vi "Add HTML Documentation for VI's parent item.vi"(11 "error in (no error)":errorcluster) -> (15 "error out":errorcluster)   [LabVIEW 2012]
doc: "VI Description text"
uses:
  _Controls and TypeDefs/InfoFromOldHTML_cluster.ctl
  _Controls and TypeDefs/StartPathLocation_enum.ctl
  _Controls and TypeDefs/UserDialogStates.ctl
  <vilib>/Platform/browser.llb/Open URL in Default Browser (string).vi
  <vilib>/Platform/browser.llb/Open URL in Default Browser (path).vi
panel:
  in  "www.labicom.net":bool
  in  "_vi_name_":string caption="Name"
  in  "Table":string[][](table)=[[" "]]
  in  "Help Button":bool
  out "LV <help> directory?":bool
  in  "Info extracted from old HTML":T1={"_vi_name_"="", "_vi_description_text_"="", "_vi_controls_and_indicators_descriptions_"="", "_name_of_owning_library_"="", "_owning_library_html_"="", "_Packages_"="Base Package", "_Platforms_"="Windows", "_details_text_"="Put details here", "_example_screenshot_"="", "_example_vi_"="", "_path_to_example_file_"=path "", "IsDetailsON?"=FALSE, "IsOwningLibraryON?"=FALSE, "IsExamplesON?"=FALSE, "IsTableON?"=FALSE, "IsScrollableON?"=FALSE, "IsDetailedHelpLinkON?"=FALSE, "Table Objects array"=[], "Table Descriptions array"=[], "Table Links array"=[], "Start path location"=enum."VI folder"}
  in  "Next_btn":bool
  out "HTML File Path":path
  in  "Cancel Button":bool
  out "Cancelled by User?":bool
  in  "Examples_chkBox":bool=TRUE
  in  "Details_chkBox":bool=TRUE
  in  "OwningLibrary_chkBox":bool=TRUE
  in  "Name of Owning Library":string="Put a name here" caption="Name of Owning Library or Palette"
  in  "Path to Owning Library":string caption="Path to Owning Library or Palette"
  in  "Names of Packages":string="Base Package" caption="Names of libraries/packages that this item requires for its operation"
  in  "Names of Platforms":string="Windows" caption="Names of platforms that this item supports"
  in  "Details":string="Put details here"
  in  "Image Path for Example":string caption="Path to the image file for Example category"
  in  "Example VI name":string
  in  "Example VI Path":path
  in  "VI Description":string caption="Item Description (with HTML tags)"
  in  "Start path location":enum32{"VI folder", "Help folder"}(radio)
  in  "Documentable VI Path":path
  # "Configure parent item Documentation Layout"
  # "Additional layout elements for LabVIEW help"
  # "Caution: place <_caution_> into your text"
  # "Note: place <_note_> into your text"
  # "Tip: place <_tip_> into your text"
  # "Windows"
  # "Platform: enclose platform name between\n<_platform_> and </_platform_> tags"
  # "bold"
  # "Text in bold: enclose such text between\n<B> and </B> tags"
  # "Attention!"
  # "Caution Text: enclose such text between \n<_caution_text_> and </_caution_text_> tags"
  # "vigods.com"
  # "Link: place path in place of '_path_' and text in \nplace of '_text_' and insert resulting string\nwherever you need: \n<a href=\"_path_\">_text_</a>"
  # "monospace"
  # "Monospace: enclose such text between\n<_monospace_> and </_monospace_> tags"
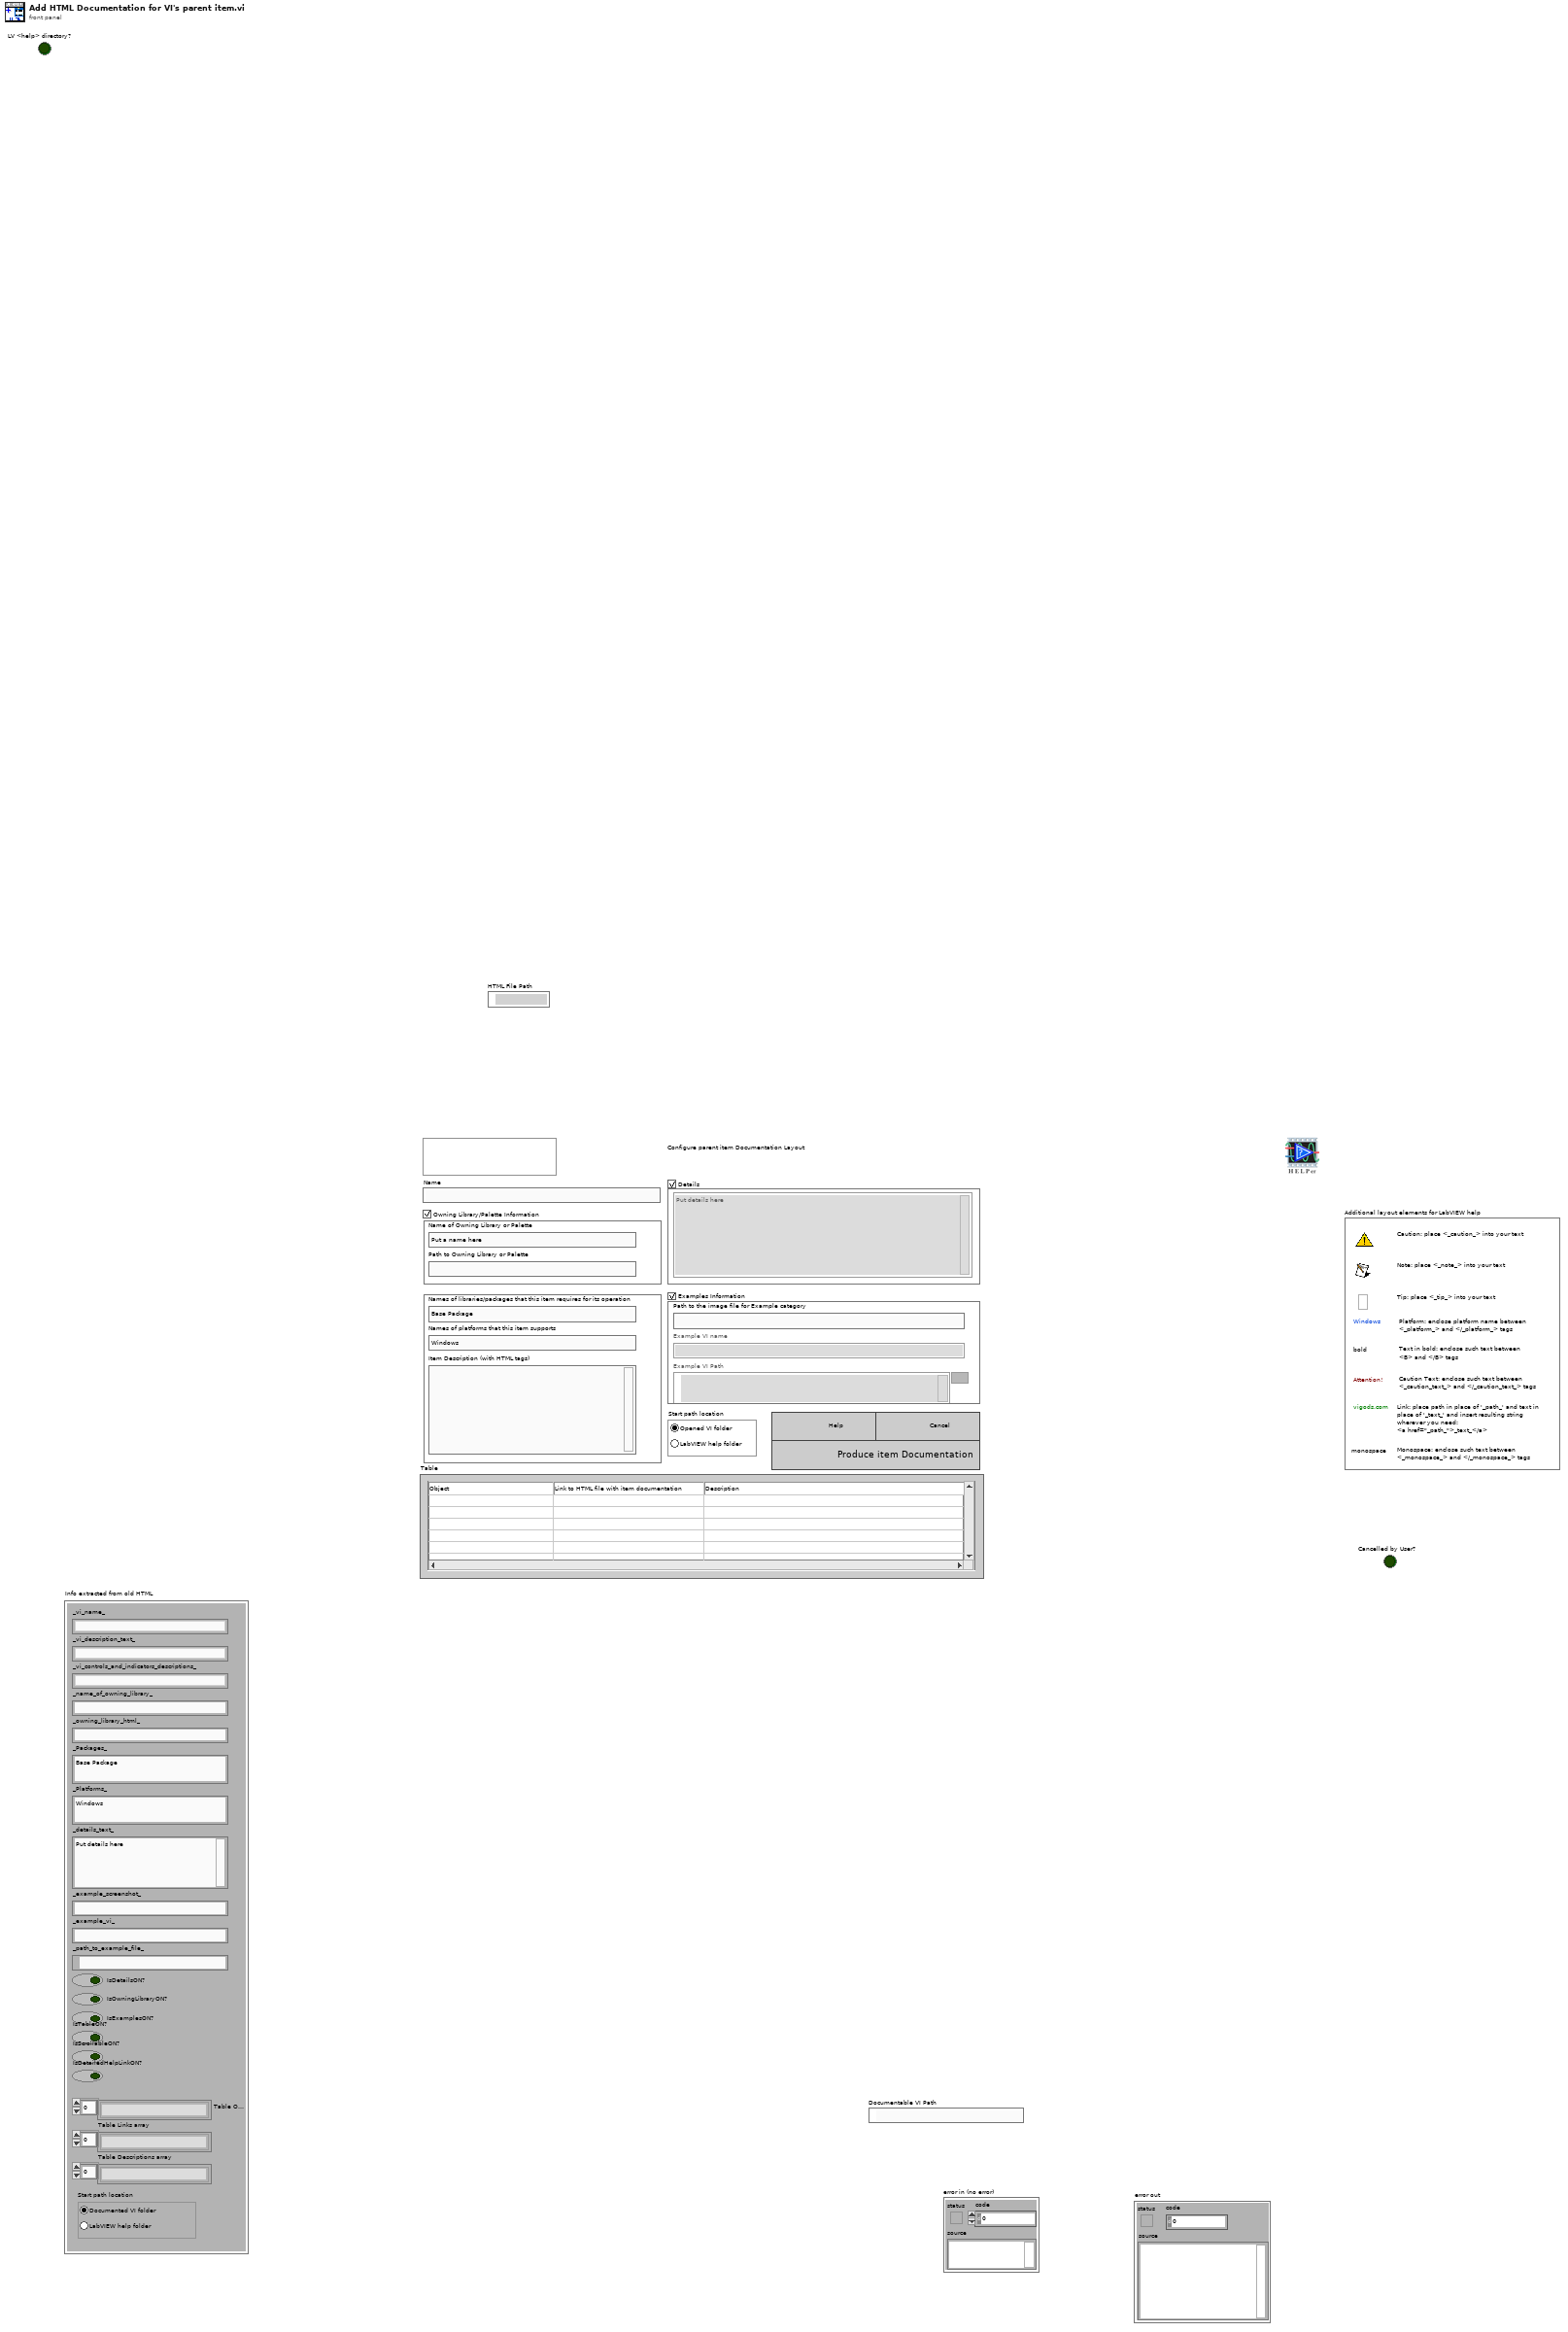
[diagram p1: front panel]
types:
  T1 = typedef "InfoFromOldHTML_cluster.ctl" = cluster{"_vi_name_":string, "_vi_description_text_":string, "_vi_controls_and_indicators_descriptions_":string, "_name_of_owning_library_":string, "_owning_library_html_":string, "_Packages_":string, "_Platforms_":string, "_details_text_":string, "_example_screenshot_":string, "_example_vi_":string, "_path_to_example_file_":path, "IsDetailsON?":bool, "IsOwningLibraryON?":bool, "IsExamplesON?":bool, "IsTableON?":bool, "IsScrollableON?":bool, "IsDetailedHelpLinkON?":bool, "Table Objects array":string[], "Table Descriptions array":string[], "Table Links array":string[], "Start path location":T2}
  T2 = typedef "StartPathLocation_enum.ctl" = enum32{"VI folder", "Help folder"}
  T3 = typedef "UserDialogStates.ctl" = enum16{"Overview", "Known Issues", "Choose parameters", "Update", "Choose HTML file path", "Choose Images directory path", "Decide if there is Context Help", "Choose help hierarchy", "Generate HTML", "Installation", "System Requirements", "Software Support", "Device Support", "Upgrade Issues", "New Features", "Fixed Issues", "Developer", "Contact Support", "Copyright", "Trademarks", "Patents", "Disclaimer", "Save", "Shutdown"}
  T4 = enum8{"Enabled", "Disabled", "Disabled and Grayed Out"}
  T5 = typedef "LVRowAndColumnTypeDef.ctl" = cluster{"Row":i32, "Column":i32}
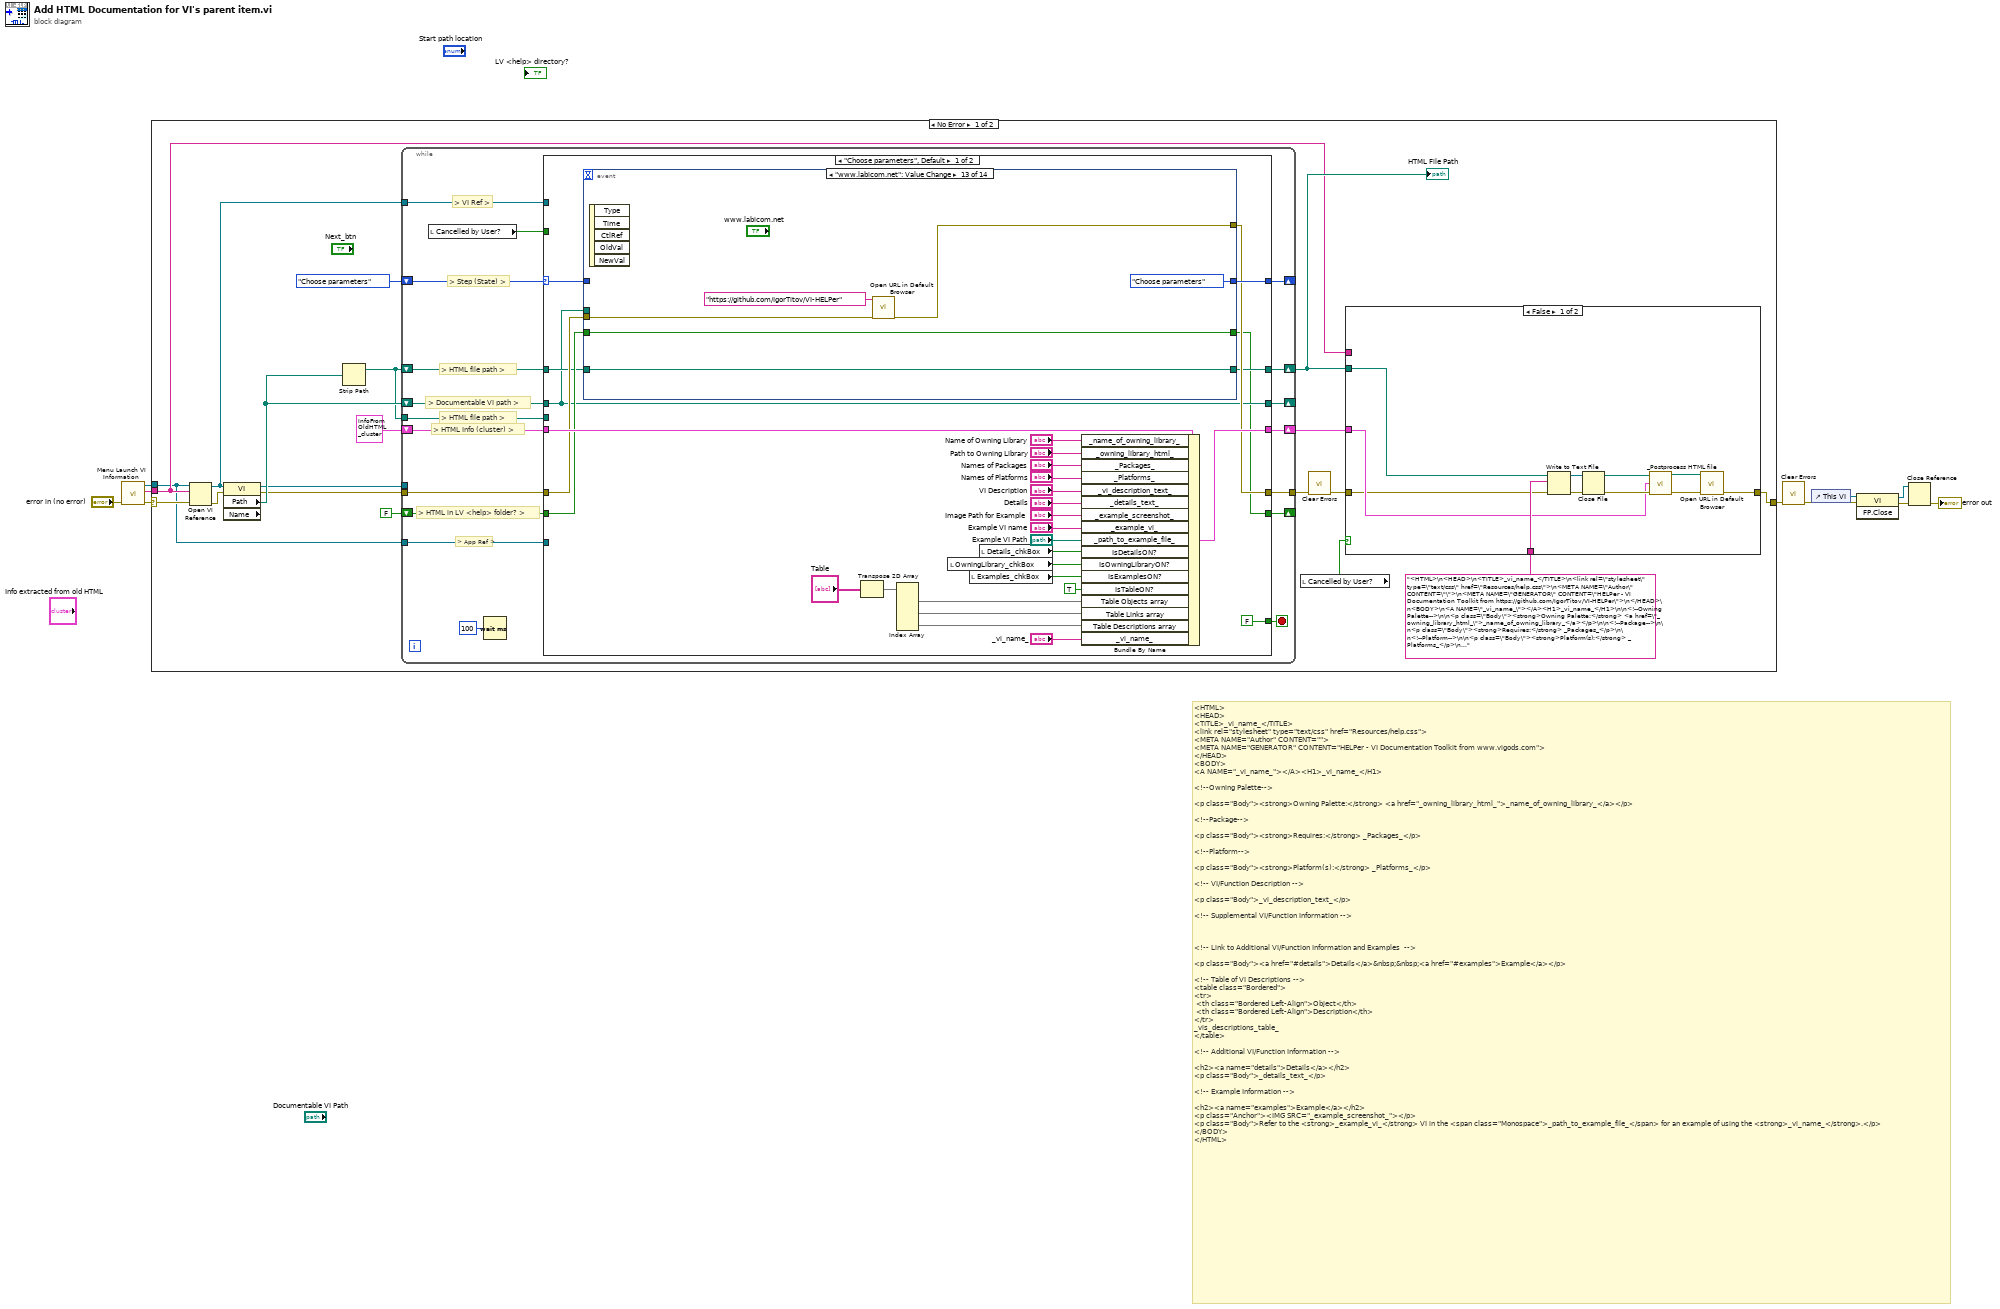
[diagram p0: block diagram]
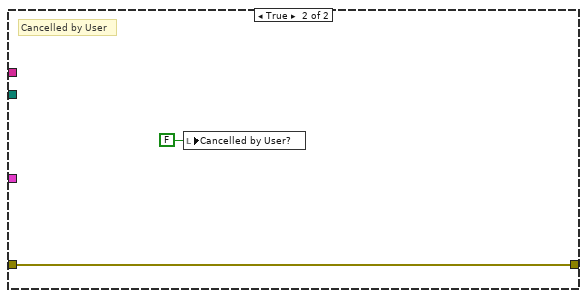
[diagram p2: hidden frame]
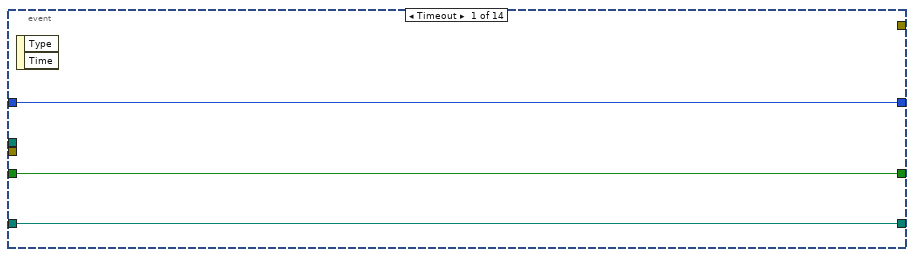
[diagram p3: hidden frame]
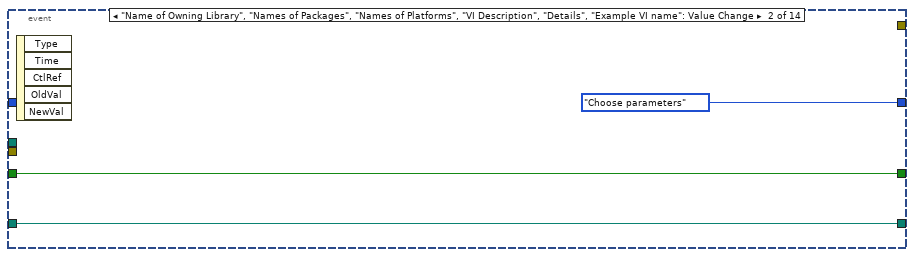
[diagram p4: hidden frame]
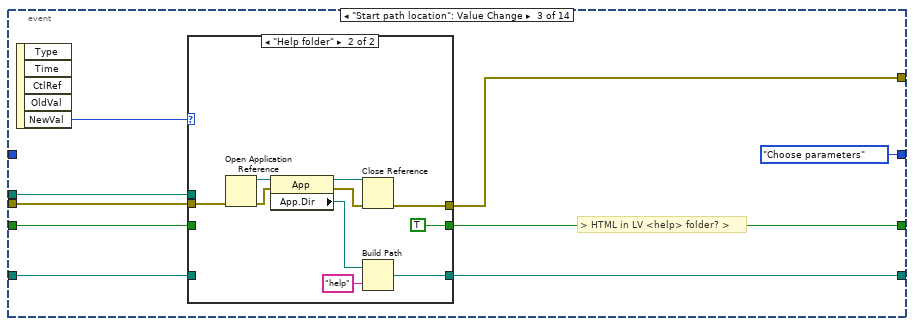
[diagram p5: hidden frame]
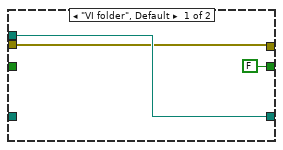
[diagram p6: hidden frame]
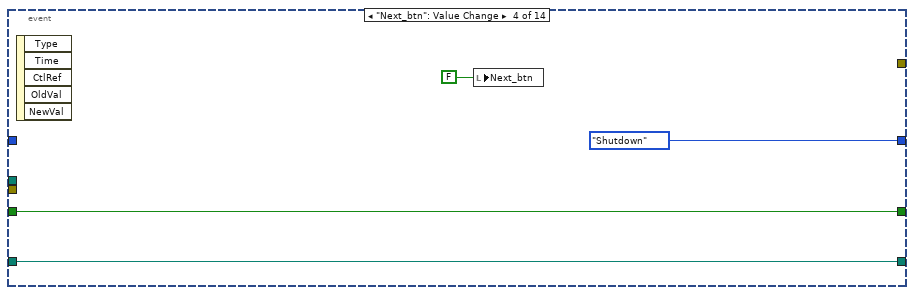
[diagram p7: hidden frame]
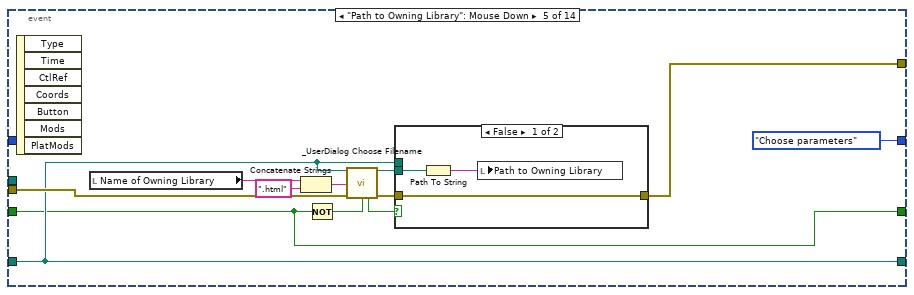
[diagram p8: hidden frame]
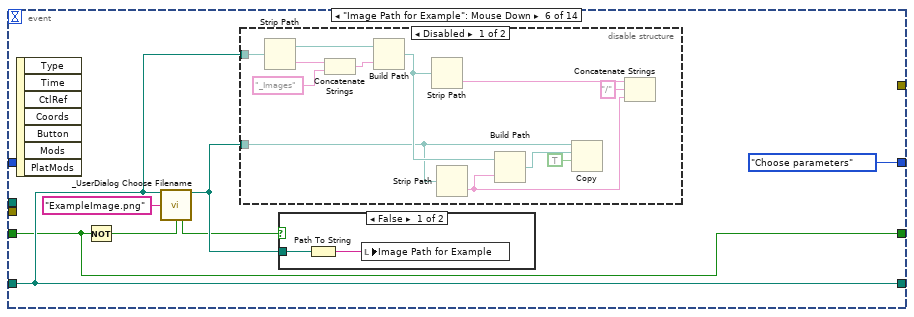
[diagram p10: hidden frame]
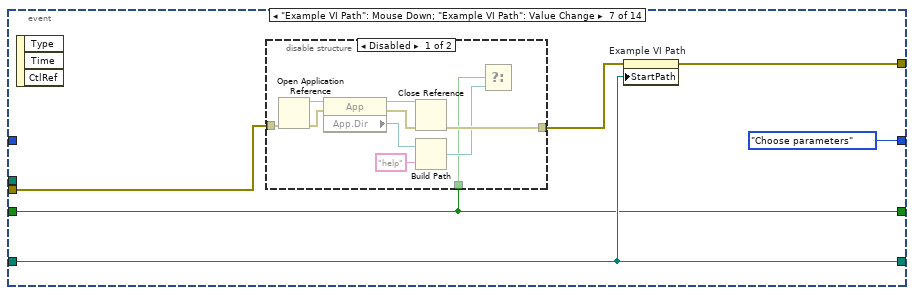
[diagram p13: hidden frame]
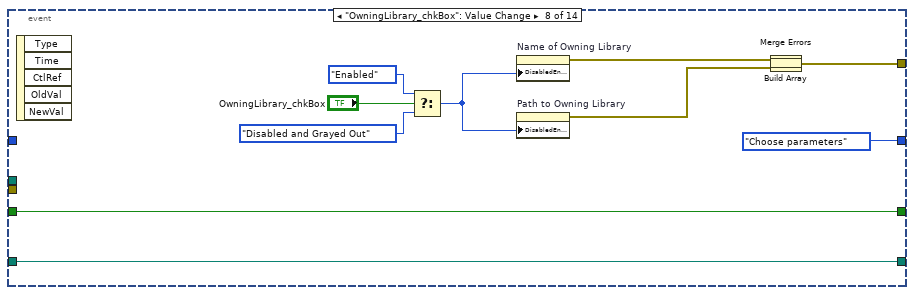
[diagram p15: hidden frame]
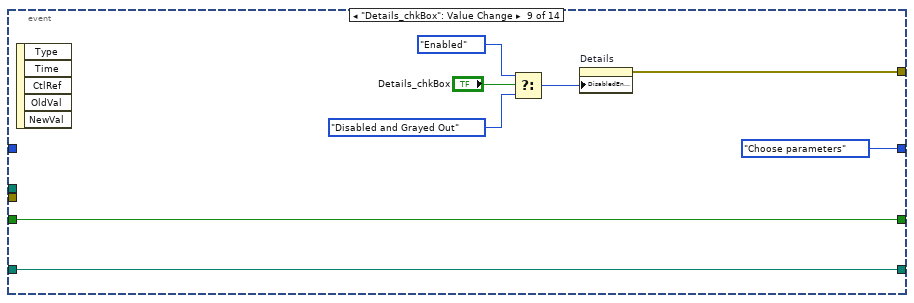
[diagram p16: hidden frame]
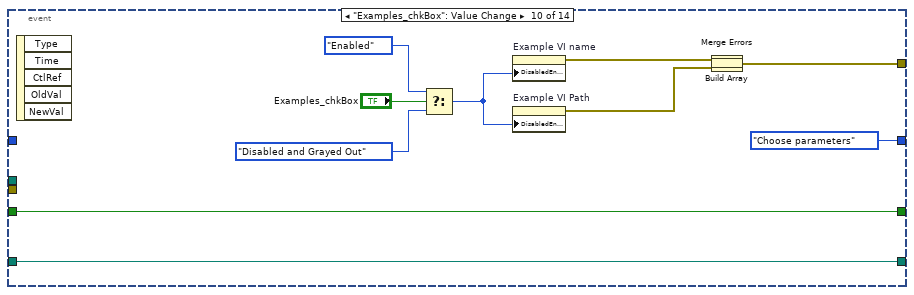
[diagram p17: hidden frame]
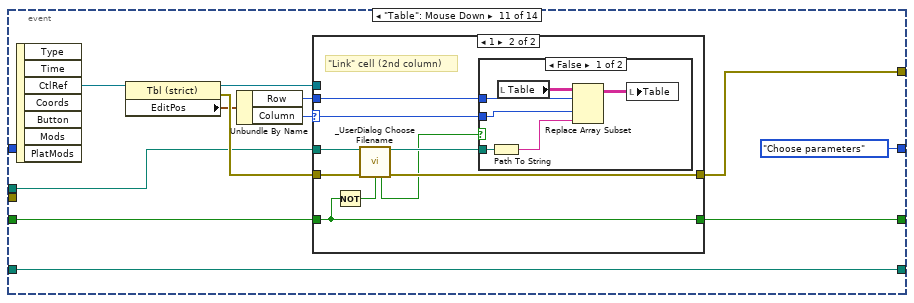
[diagram p18: hidden frame]
diagram:
  # "<HTML>\n<HEAD>\n<TITLE>_vi_name_</TITLE>\n<link rel=\"stylesheet\" type=\"text/css\" href=\"Resources/help.css\">\n<META NAME=\"Author\" CONTENT=\"\">\n<META NAME=\"GENERATOR\" CONTENT=\"HELPer - VI Documentation Toolkit from www.vigods.com\">\n</HEAD>\n<BODY>\n<A NAME=\"_vi_name_\"></A><H1>_vi_name_</H1>\n\n<!--Owning Palette-->\n\n<p class=\"Body\"><strong>Owning Palette:</strong> <a href=\"_owning_library_html_\">_name_of_owning_library_</a></p>\n\n<!--Package-->\n\n<p class=\"Body\"><strong>Requires:</strong> _Packages_</p>\n\n<!--Platform-->\n\n<p class=\"Body\"><strong>Platform(s):</strong> _Platforms_</p>\n\n<!-- VI/Function Description -->\n\n<p class=\"Body\">_vi_description_text_</p>\n\n<!-- Supplemental VI/Function Information -->\n\n\n\n<!-- Link to Additional VI/Function Information and Examples  -->\n\n<p class=\"Body\"><a href=\"#details\">Details</a>&nbsp;&nbsp;<a href=\"#examples\">Example</a></p>\n\n<!-- Table of VI Descriptions -->\n<table class=\"Bordered\">\n<tr>\n\t<th class=\"Bordered Left-Align\">Object</th>\n\t<th class=\"Bordered Left-Align\">Description</th>\n</tr>\n_vis_descriptions_table_\n</table>\n\n<!-- Additional VI/Function Information -->\n\n<h2><a name=\"details\">Details</a></h2>\n<p class=\"Body\">_details_text_</p>\n\n<!-- Example Information -->\n\n<h2><a name=\"examples\">Example</a></h2>\n<p class=\"Anchor\"><IMG SRC=\"_example_screenshot_\"></p>\n<p class=\"Body\">Refer to the <strong>_example_vi_</strong> VI in the <span class=\"Monospace\">_path_to_example_file_</span> for an example of using the <strong>_vi_name_</strong>.</p>\n</BODY>\n</HTML>"
  n1 = call <vilib>:"Menu Launch VI Information.vi"("error in (no error)"="error in (no error)") -> ("error out"=w7:errorcluster, "Menu Launch:VI"=w9:string, "Menu Launch:App"=w10:refnum<vi>)  [unwired: 8 in]
  n2 = case shown="No Error" w7 {
    selector: w7 -> [w26 w350]
    tunnel: w10 -> [w17 _]
    tunnel: w9 -> [w18 _]
    tunnel: [w23 w350] -> w2
    frame No Error {
      n3 = Open VI Reference(application reference (local)=w17, vi path=w18, error in (no error)=w26) -> (vi reference=w19:refnum<vi>, error out=w29:errorcluster)  [unwired: 3 in]
      n4 = property class="VI" props=["Path", "Name"](reference=w19, error in=w29) -> (reference out=w15:refnum<vi>, error out=w16:errorcluster, "Path"=w21:path)  [unwired: 1 out]
      n5 = Strip Path(path=w21) -> (stripped path=w20:path)  [unwired: 1 out]
      n6 = while {
        shift-right: [w57] -> _
        shift-left: UserDialogStates."Choose parameters" ("UserDialogSteps") -> [w58]
        tunnel: w20 -> [w56]
        shift-right: [w55] -> w22
        shift-left: w20 -> [w54]
        shift-right: [w52] -> w24
        shift-left: T1 {"_vi_name_"="", "_vi_description_text_"="", "_vi_controls_and_indicators_descriptions_"="", "_name_of_owning_library_"="", "_owning_library_html_"="", "_Packages_"="Base Package", "_Platforms_"="Windows", "_details_text_"="Put details here", "_example_screenshot_"="", "_example_vi_"="", "_path_to_example_file_"=path "", "IsDetailsON?"=FALSE, "IsOwningLibraryON?"=FALSE, "IsExamplesON?"=FALSE, "IsTableON?"=FALSE, "IsScrollableON?"=FALSE, "IsDetailedHelpLinkON?"=FALSE, "Table Objects array"=[], "Table Descriptions array"=[], "Table Links array"=[], "Start path location"=enum."VI folder"} ("Info extracted from old HTML") -> [w53]
        tunnel: w16 -> [w50]
        shift-right: [w47] -> _
        shift-left: FALSE -> [w51]
        shift-right: [w46] -> _
        shift-left: w21 -> [w49]
        tunnel: [w48] -> w12
        tunnel: w19 -> [w44]
        tunnel: w17 -> [w43]
        tunnel: w15 -> [_]
        stop <- w60 stop-if-true
        # "> App Ref >"
        # "> VI Ref >"
        # "> Documentable VI path >"
        # "> HTML file path >"
        # "> HTML in LV <help> folder? >"
        # "> HTML Info (cluster) >"
        # "> Step (State) >"
        # "> HTML file path >"
        n7 = local read "Cancelled by User?"() -> (w45:bool)
        n8 = Wait (ms)(milliseconds to wait=u32 100) -> ()  [unwired: 1 out]
        n9 = case shown="\"Choose parameters\", Default" w58 {
          selector: w58 -> [w90 w256]
          tunnel: [FALSE w269] -> w60
          tunnel: [w89 w262] -> w57
          tunnel: w56 -> [_ _]
          tunnel: [w70 w260] -> w55
          tunnel: w54 -> [w71 w263]
          tunnel: w53 -> [w88 w266]
          tunnel: [w78 w265] -> w52
          tunnel: w51 -> [w72 w259]
          tunnel: w50 -> [w74 w268]
          tunnel: w49 -> [w69 w267]
          tunnel: [w73 w264] -> w48
          tunnel: [w68 w258] -> w47
          tunnel: [w69 w261] -> w46
          tunnel: w45 -> [_ w257]
          tunnel: w44 -> [_ w255]
          tunnel: w43 -> [_ w254]
          frame "Choose parameters", Default {
            n10 = event shown="[12] \"www.labicom.net\": Value Change" {
              selector: _ -> [_ _ _ _ _ _ _ _ _ _ _ _ _ _]
              dyn-events: _ -> [_ _ _ _ _ _ _ _ _ _ _ _ _ _]
              timeout: _ -> [_ _ _ _ _ _ _ _ _ _ _ _ _ _]
              tunnel: w90 -> [w94 _ _ _ _ _ _ _ _ _ _ _ _ _]
              tunnel: [w94 UserDialogStates."Choose parameters" ("UserDialogSteps") UserDialogStates."Choose parameters" ("UserDialogSteps") UserDialogStates."Shutdown" ("UserDialogSteps") UserDialogStates."Choose parameters" ("UserDialogSteps") UserDialogStates."Choose parameters" ("UserDialogSteps") UserDialogStates."Choose parameters" ("UserDialogSteps") UserDialogStates."Choose parameters" ("UserDialogSteps") UserDialogStates."Choose parameters" ("UserDialogSteps") UserDialogStates."Choose parameters" ("UserDialogSteps") UserDialogStates."Choose parameters" ("UserDialogSteps") UserDialogStates."Choose parameters" ("UserDialogSteps") UserDialogStates."Choose parameters" ("UserDialogSteps") UserDialogStates."Shutdown" ("UserDialogSteps")] -> w89
              tunnel: w72 -> [w92 w95 w99 w120 w124 w140 w161 w179 w189 w198 w213 w241 w244 w249]
              tunnel: w74 -> [_ _ w102 _ w129 _ w164 _ _ _ _ w238 w247 w252]
              tunnel: [_ _ w101 _ w128 _ w163 w180 w191 w200 w211 w237 w246 w252] -> w73
              tunnel: w71 -> [w93 w96 w104 w121 w127 w144 w162 w183 w190 w199 w212 w240 w245 w250]
              tunnel: [w93 w96 w103 w121 w127 w144 w162 w183 w190 w199 w212 w240 w245 w250] -> w70
              tunnel: w69 -> [_ _ w100 _ _ _ _ _ _ _ w214 _ _ _]
              tunnel: [w92 w95 w98 w120 w124 w140 w161 w179 w189 w198 w208 w241 w244 w249] -> w68
              event Timeout {
                n11 = event-data() -> ()  [unwired: 1 in, 2 out]
              }
              event "Name of Owning Library", "Names of Packages", "Names of Platforms", "VI Description", "Details", "Example VI name": Value Change {
                n12 = event-data() -> ()  [unwired: 1 in, 5 out]
              }
              event "Start path location": Value Change {
                # "> HTML in LV <help> folder? >"
                n13 = event-data() -> ("NewVal"=w105:enum32{"VI folder", "Help folder"})  [unwired: 1 in, 4 out]
                n14 = case shown="\"Help folder\"" w105 {
                  tunnel: w104 -> [_ _]
                  tunnel: [w109 w113] -> w103
                  tunnel: w102 -> [w108 w112]
                  tunnel: [w108 w111] -> w101
                  tunnel: w100 -> [w109 _]
                  tunnel: w99 -> [_ _]
                  tunnel: [FALSE TRUE] -> w98
                  frame "VI folder", Default {
                  }
                  frame "Help folder" {
                    n15 = Open Application Reference(8:w112) -> (0:w115:errorcluster, 3:w114:refnum<vi>)  [unwired: 3 in]
                    n16 = property class="App"(reference=w114, error in=w115) -> (reference out=w116:refnum<vi>, error out=w117:errorcluster, "App.Dir"=w118:path)
                    n17 = Close Reference(reference=w116, error in (no error)=w117) -> (error out=w111:errorcluster)
                    n18 = Build Path(base path=w118, name or relative path="help") -> (appended path=w113:path)
                  }
                }
              }
              event "Next_btn": Value Change {
                n19 = event-data() -> ()  [unwired: 1 in, 5 out]
                n20 = local write "Next_btn"(FALSE ("Next Button")) -> ()
              }
              event "Path to Owning Library": Mouse Down {
                n21 = event-data() -> ()  [unwired: 1 in, 7 out]
                n22 = local read "Name of Owning Library"() -> (w134:string)
                n23 = Concatenate Strings(w134, ".html" ("string")) -> (w133:string)
                n24 = Not(x=w124) -> (.not. x?=w125:bool)
                n25 = call "_UserDialog Choose Filename.vi"("VI Default Path"=w127, "Default file name"=w133, "error in (no error)"=w129, "Not In <help> directory? (Yes: T)"=w125) -> ("HTML File Path"=w131:path, "Cancelled by User?"=w126:bool, "error out"=w130:errorcluster)  [unwired: 7 in, 2 out]
                n26 = case shown="False" w126 {
                  tunnel: w131 -> [w138 _]
                  tunnel: w130 -> [w136 w139]
                  tunnel: [w136 w139] -> w128
                  tunnel: w127 -> [_ _]
                  frame False {
                    n27 = Path To String(path=w138) -> (string=w137:string)
                    n28 = local write "Path to Owning Library"(w137) -> ()
                  }
                  frame True {
                  }
                }
              }
              event "Image Path for Example": Mouse Down {
                n29 = event-data() -> ()  [unwired: 1 in, 7 out]
                n30 = Not(x=w140) -> (.not. x?=w141:bool)
                n31 = call "_UserDialog Choose Filename.vi"("VI Default Path"=w144, "Default file name"="ExampleImage.png", "Not In <help> directory? (Yes: T)"=w141) -> ("HTML File Path"=w143:path, "Cancelled by User?"=w142:bool)  [unwired: 8 in, 3 out]
                n32 = disable-structure shown="Disabled" {
                  disable-tunnel: w144 -> [w148 _]
                  disable-tunnel: w143 -> [w147 _]
                  frame Disabled {
                    n33 = Strip Path(path=w148) -> (stripped path=w150:path, name=w152:string)
                    n34 = Concatenate Strings(w152, "_Images" ("name or relative path")) -> (w153:string)
                    n35 = Build Path(base path=w150, name or relative path=w153) -> (appended path=w149:path)
                    n36 = Strip Path(path=w149) -> (name=w156:string)  [unwired: 1 out]
                    n37 = Strip Path(path=w147) -> (name=w155:string)  [unwired: 1 out]
                    n38 = Build Path(base path=w149, name or relative path=w155) -> (appended path=w158:path)
                    n39 = Copy(9:TRUE ("overwrite (F)"), 10:w158, 11:w147) -> ()  [unwired: 2 in, 3 out]
                    n40 = Concatenate Strings(w156, "/" ("string"), w155) -> ()  [unwired: 1 out]
                  }
                  frame Enabled {
                  }
                }
                n41 = case shown="False" w142 {
                  tunnel: w143 -> [w160 _]
                  frame False {
                    n42 = Path To String(path=w160) -> (string=w159:string)
                    n43 = local write "Image Path for Example"(w159) -> ()
                  }
                  frame True {
                  }
                }
              }
              event "Example VI Path": Mouse Down; "Example VI Path": Value Change {
                n44 = event-data() -> ()  [unwired: 1 in, 3 out]
                n45 = disable-structure shown="Disabled" {
                  disable-tunnel: [w176 w177] -> w165
                  disable-tunnel: w161 -> [w168 _]
                  disable-tunnel: w164 -> [w167 w177]
                  frame Disabled {
                    n46 = Open Application Reference(8:w167) -> (0:w173:errorcluster, 3:w174:refnum<vi>)  [unwired: 3 in]
                    n47 = property class="App"(reference=w174, error in=w173) -> (reference out=w172:refnum<vi>, error out=w171:errorcluster, "App.Dir"=w170:path)
                    n48 = Close Reference(reference=w172, error in (no error)=w171) -> (error out=w176:errorcluster)
                    n49 = Build Path(base path=w170, name or relative path="help") -> (appended path=w175:path)
                    n50 = Select(s=w168, f=w175) -> ()  [unwired: 1 in, 1 out]
                  }
                  frame Enabled {
                  }
                }
                n51 = property on="Example VI Path" class="Path"(error in=w165, "StartPath"=w162) -> (error out=w163:errorcluster)  [unwired: 1 in, 1 out]
              }
              event "OwningLibrary_chkBox": Value Change {
                n52 = event-data() -> ()  [unwired: 1 in, 5 out]
                n53 = Select(t=T4."Enabled" ("Disabled"), s="OwningLibrary_chkBox", f=T4."Disabled and Grayed Out") -> (s? t:f=w184:T4)
                n54 = property on="Name of Owning Library" class="Str"("DisabledEnum"=w184) -> (error out=w182:errorcluster)  [unwired: 2 in, 1 out]
                n55 = property on="Path to Owning Library" class="Str"("DisabledEnum"=w184) -> (error out=w181:errorcluster)  [unwired: 2 in, 1 out]
                n56 = Build Array(w182, w181) -> (w178:errorcluster[])
                n57 = Merge Errors(w178) -> (w180:errorcluster)
              }
              event "Details_chkBox": Value Change {
                n58 = event-data() -> ()  [unwired: 1 in, 5 out]
                n59 = Select(t=T4."Enabled" ("Disabled"), s="Details_chkBox", f=T4."Disabled and Grayed Out") -> (s? t:f=w194:T4)
                n60 = property on="Details" class="Str"("DisabledEnum"=w194) -> (error out=w191:errorcluster)  [unwired: 2 in, 1 out]
              }
              event "Examples_chkBox": Value Change {
                n61 = event-data() -> ()  [unwired: 1 in, 5 out]
                n62 = Select(t=T4."Enabled" ("Disabled"), s="Examples_chkBox", f=T4."Disabled and Grayed Out") -> (s? t:f=w204:T4)
                n63 = property on="Example VI name" class="Str"("DisabledEnum"=w204) -> (error out=w202:errorcluster)  [unwired: 2 in, 1 out]
                n64 = property on="Example VI Path" class="Path"("DisabledEnum"=w204) -> (error out=w201:errorcluster)  [unwired: 2 in, 1 out]
                n65 = Build Array(w202, w201) -> (w197:errorcluster[])
                n66 = Merge Errors(w197) -> (w200:errorcluster)
              }
              event "Table": Mouse Down {
                n67 = event-data() -> ("CtlRef"=w210:refnum<vi>)  [unwired: 1 in, 6 out]
                n68 = property class="Tbl (strict)"(reference=w210) -> (reference out=w217:refnum<vi>, error out=w218:errorcluster, "EditPos"=w215:T5)  [unwired: 1 in]
                n69 = Unbundle By Name(w215) -> ("Row"=w219:i32, "Column"=w216:i32)
                n70 = case shown="1" w216 {
                  selector: w216 -> [_ w226]
                  tunnel: w213 -> [w220 w224]
                  tunnel: w214 -> [_ w230]
                  tunnel: w217 -> [_ _]
                  tunnel: w218 -> [w221 w228]
                  tunnel: w219 -> [_ w227]
                  tunnel: [w221 w225] -> w211
                  tunnel: [w220 w224] -> w208
                  frame 0, Default {
                  }
                  frame 1 {
                    # "\"Link\" cell (2nd column)"
                    n71 = Not(x=w224) -> (.not. x?=w223:bool)
                    n72 = call "_UserDialog Choose Filename.vi"("VI Default Path"=w230, "error in (no error)"=w228, "Not In <help> directory? (Yes: T)"=w223) -> ("HTML File Path"=w229:path, "Cancelled by User?"=w222:bool, "error out"=w225:errorcluster)  [unwired: 8 in, 2 out]
                    n73 = case shown="False" w222 {
                      tunnel: w229 -> [w236 _]
                      tunnel: w227 -> [w234 _]
                      tunnel: w226 -> [w233 _]
                      frame False {
                        n74 = Path To String(path=w236) -> (string=w232:string)
                        n75 = local read "Table"() -> (w235:string[][])
                        n76 = Replace Array Subset(array=w235, new element=w232, index (row)=w234, index (col)=w233) -> (w231:string[][])
                        n77 = local write "Table"(w231) -> ()
                      }
                      frame True {
                      }
                    }
                  }
                }
              }
              event "Help Button": Value Change {
                n78 = event-data() -> ()  [unwired: 1 in, 5 out]
                n79 = call "Read me and Help.vi"("path"=path "viGods.com/HELPer/parent.html", "error in"=w238) -> ("error out"=w237:errorcluster)  [unwired: 13 in]
              }
              event "www.labicom.net": Value Change {
                n80 = event-data() -> ()  [unwired: 1 in, 5 out]
                n81 = call-poly <vilib>:"Open URL in Default Browser.vi"("error in (no error)"=w247, "URL"="https://github.com/IgorTitov/VI-HELPer") -> ("error out"=w246:errorcluster)  [unwired: 4 in, 1 out]
              }
              event "Cancel Button": Value Change {
                n82 = event-data() -> ()  [unwired: 1 in, 5 out]
                "Cancelled by User?" <- TRUE ("Cancelled by User?")
              }
            }
            n83 = Transpose 2D Array(2D array="Table") -> (transposed array=w62:string[][])
            n84 = Index Array(array=w62) -> (element #1=w66:string[], element #2=w65:string[], element #3=w64:string[])  [unwired: 6 in]
            n85 = local read "OwningLibrary_chkBox"() -> (w76:bool)
            n86 = local read "Examples_chkBox"() -> (w75:bool)
            n87 = local read "Details_chkBox"() -> (w77:bool)
            n88 = Bundle By Name(cluster=w88, "_name_of_owning_library_"="Name of Owning Library", "_owning_library_html_"="Path to Owning Library", "_Packages_"="Names of Packages", "_Platforms_"="Names of Platforms", "_vi_description_text_"="VI Description", "_details_text_"="Details", "_example_screenshot_"="Image Path for Example", "_example_vi_"="Example VI name", "_path_to_example_file_"="Example VI Path", "IsDetailsON?"=w77, "IsOwningLibraryON?"=w76, "IsExamplesON?"=w75, "IsTableON?"=TRUE, "Table Objects array"=w66, "Table Links array"=w65, "Table Descriptions array"=w64, "_vi_name_"="_vi_name_") -> (w78:T1)
          }
          frame "Shutdown" {
            n89 = case shown="False" w257 {
              tunnel: [w289 TRUE] -> w269
              tunnel: w268 -> [w288 w342]
              tunnel: w267 -> [w287 w345]
              tunnel: w266 -> [w286 w346]
              tunnel: [w285 w346] -> w265
              tunnel: [w284 w341] -> w264
              tunnel: w263 -> [w283 w344]
              tunnel: [w281 UserDialogStates."Shutdown" ("UserDialogSteps")] -> w262
              tunnel: [w280 w345] -> w261
              tunnel: [w279 w344] -> w260
              tunnel: w259 -> [w276 w347]
              tunnel: [w277 w347] -> w258
              tunnel: w256 -> [_ _]
              tunnel: w255 -> [w272 w343]
              tunnel: w254 -> [w271 _]
              frame False {
                # "> VI Name >"
                n90 = Concatenate Strings("parent_item" ("string"), ".html" ("string")) -> (w273:string)
                n91 = Not(x=w276) -> (.not. x?=w275:bool)
                n92 = call "_UserDialog Choose Filename.vi"("VI Default Path"=w283, "Default file name"=w273, "Not In <help> directory? (Yes: T)"=w275) -> ("HTML File Path"=w282:path, "Cancelled by User?"=w278:bool)  [unwired: 8 in, 3 out]
                n93 = case shown="False" w278 {
                  tunnel: [TRUE FALSE] -> w289
                  tunnel: w288 -> [w293 w338]
                  tunnel: w287 -> [w302 w335]
                  tunnel: w286 -> [w317 w336]
                  tunnel: [w315 w336] -> w285
                  tunnel: [w313 w338] -> w284
                  tunnel: w282 -> [w295 w334]
                  tunnel: [UserDialogStates."Shutdown" ("UserDialogSteps") UserDialogStates."Choose parameters" ("UserDialogSteps")] -> w281
                  tunnel: [w302 w335] -> w280
                  tunnel: [w295 w334] -> w279
                  tunnel: w276 -> [w303 w337]
                  tunnel: [w303 w337] -> w277
                  tunnel: w272 -> [w298 _]
                  tunnel: w271 -> [_ _]
                  frame False {
                    # "Copy example image from location chosen by user\nto images folder of this HTML"
                    # "> HTML file path >"
                    # "> Documented VI path >"
                    # "> HTML file path >"
                    n94 = Unbundle By Name(w317) -> ("_owning_library_html_"=w323:string, "_example_screenshot_"=w307:string, "Table Links array"=w301:string[])
                    n95 = call "_Create HTML folders.vi"("HTML File Path"=w295, "error in (no error)"=w293) -> ("HTML Images Folder"=w292:path, "error out"=w294:errorcluster)  [unwired: 10 in, 2 out]
                    n96 = String To Path(string=w323) -> (path=w318:path)
                    n97 = String To Path(string=w307) -> (path=w306:path)
                    n98 = String To Path(string=w301) -> (path=w300:path[])
                    n99 = for {
                      tunnel: w300 -> [w328] mode=indexing
                      tunnel: w295 -> [w329]
                      tunnel: [w325] -> w299 mode=indexing
                      tunnel: w294 -> [w326]
                      tunnel: [w327] -> w296
                      n100 = call <vilib>:"Compare Two Paths.vi"("error in (no error)"=w326, "Path 2"=w328, "Path 1"=w329) -> ("error out"=w330:errorcluster, "Relative Path from 1 to 2"=w331:path)  [unwired: 5 in, 2 out]
                      n101 = Path To String(path=w331) -> (string=w332:string)
                      n102 = Search and Replace String(input string=w332, search string="..\\", error in=w330) -> (result string=w325:string, error out=w327:errorcluster)  [unwired: 5 in, 2 out]
                    }
                    n103 = call <vilib>:"Compare Two Paths.vi"("error in (no error)"=w294, "Path 2"=w318, "Path 1"=w295) -> ("error out"=w322:errorcluster, "Relative Path from 1 to 2"=w321:path)  [unwired: 5 in, 2 out]
                    n104 = Path To String(path=w321) -> (string=w320:string)
                    n105 = Strip Path(path=w306) -> (name=w311:string)  [unwired: 1 out]
                    n106 = Strip Path(path=w292) -> (name=w310:string)  [unwired: 1 out]
                    n107 = Search and Replace String(input string=w320, search string="..\\", error in=w322) -> (result string=w316:string, error out=w297:errorcluster)  [unwired: 5 in, 2 out]
                    n108 = Build Path(base path=w292, name or relative path=w311) -> (appended path=w308:path)
                    n109 = Copy(8:w297, 9:TRUE ("overwrite (F)"), 10:w308, 11:w306) -> (0:w291:errorcluster)  [unwired: 1 in, 2 out]
                    n110 = Concatenate Strings(w310, "/" ("string"), w311) -> (w305:string)
                    n111 = Bundle By Name(cluster=w317, "_owning_library_html_"=w316, "_example_screenshot_"=w305, "Table Links array"=w299) -> (w315:T1)
                    n112 = Close Reference(reference=w298, error in (no error)=w297) -> (error out=w314:errorcluster)
                    n113 = Build Array(w314, w296, w291) -> (w290:errorcluster[])
                    n114 = Merge Errors(w290) -> (w313:errorcluster)
                  }
                  frame True {
                    # "Cancelled by user in the file path dialog"
                  }
                }
              }
              frame True {
                # "Cancelled by user permanently"
                n115 = Close Reference(reference=w343, error in (no error)=w342) -> (error out=w341:errorcluster)
              }
            }
          }
        }
      }
      "HTML File Path" <- w22
      n116 = local read "Cancelled by User?"() -> (w25:bool)
      n117 = call <vilib>:"Clear Errors.vi"("error in (no error)"=w12) -> ("error out"=w11:errorcluster)  [unwired: 6 in]
      n118 = case shown="False" w25 {
        tunnel: w11 -> [w33 w42]
        tunnel: w24 -> [w35 _]
        tunnel: [w30 w42] -> w23
        tunnel: "<HTML>\n<HEAD>\n<TITLE>_vi_name_</TITLE>\n<link rel=\"stylesheet\" type=\"text/css\" href=\"Resources/help.css\">\n<META NAME=\"Author\" CONTENT=\"\">\n<META NAME=\"GENERATOR\" CONTENT=\"HELPer - VI Documentation Toolkit from https://github.com/IgorTitov/VI-HELPer\">\n</HEAD>\n<BODY>\n<A NAME=\"_vi_name_\"></A><H1>_vi_name_</H1>\n\n<!--Owning Palette-->\n\n<p class=\"Body\"><strong>Owning Palette:</strong> <a href=\"_owning_library_html_\">_name_of_owning_library_</a></p>\n\n<!--Package-->\n\n<p class=\"Body\"><strong>Requires:</strong> _Packages_</p>\n\n<!--Platform-->\n\n<p class=\"Body\"><strong>Platform(s):</strong> _Platforms_</p>\n\n<!-- VI/Function Description -->\n\n<p class=\"Body\">_vi_description_text_</p>\n\n<!-- Supplemental VI/Function Information -->\n\n\n\n<!-- Link to Additional VI/Function Information and Examples  -->\n\n<p class=\"Body\"><a href=\"#details\">Details</a>&nbsp;&nbsp;<a href=\"#examples\">Example</a></p>\n\n<!-- Table of VI Descriptions -->\n<table class=\"Bordered\">\n<tr>\n\t<th class=\"Bordered Left-Align\">Object</th>\n\t<th class=\"Bordered Left-Align\">Description</th>\n</tr>\n_vis_descriptions_table_\n</table>\n\n<!-- Additional VI/Function Information -->\n\n<h2><a name=\"details\">Details</a></h2>\n<p class=\"Body\">_details_text_</p>\n\n<!-- Example Information -->\n\n<h2><a name=\"examples\">Example</a></h2>\n<p class=\"Anchor\"><IMG SRC=\"_example_screenshot_\"></p>\n<p class=\"Body\">Refer to the <strong>_example_vi_</strong> VI in the <span class=\"Monospace\">_path_to_example_file_</span> for an example of using the <strong>_vi_name_</strong>.</p>\n</BODY>\n</HTML>" -> [w37 _]
        tunnel: w22 -> [w34 _]
        tunnel: w18 -> [_ _]
        frame False {
          n119 = Write to Text File(file (use dialog)=w34, text=w37, error in=w33) -> (refnum out=w39:refnum<file>, error out=w40:errorcluster)  [unwired: 1 in, 1 out]
          n120 = Close File(refnum=w39, error in=w40) -> (path=w38:path, error out=w36:errorcluster)
          n121 = call "_Postprocess HTML file.vi"("HTML File Path"=w38, "VI Info"=w35, "error in"=w36) -> ("HTML File Path out"=w31:path, "error out"=w32:errorcluster)  [unwired: 11 in]
          n122 = call-poly <vilib>:"Open URL in Default Browser.vi"("error in (no error)"=w32, "path"=w31) -> ("error out"=w30:errorcluster)  [unwired: 4 in, 1 out]
        }
        frame True {
          # "Cancelled by User"
          n123 = local write "Cancelled by User?"(FALSE ("Cancelled by User?")) -> ()
        }
      }
    }
    frame Error {
    }
  }
  n124 = call <vilib>:"Clear Errors.vi"("error in (no error)"=w2) -> ("error out"=w3:errorcluster)  [unwired: 6 in]
  n125 = control-ref of="This VI"() -> (w6:refnum<vi>)
  n126 = invoke class="VI" method="FP.Close"(reference=w6, error in=w3) -> (reference out=w4:refnum<vi>, error out=w5:errorcluster)  [unwired: 1 in, 1 out]
  n127 = Close Reference(reference=w4, error in (no error)=w5) -> (error out=→"error out":errorcluster)
